vi "Telemetry_data_array_setup.vi"(8 "error in":errorcluster, 10 "Subsystem data":T1={"Subsystem name"="Drive", "Double data points"=[], "Boolean data points"=[], "Boolean channel names"=[], "Double channel names"=[]}, 11 "Channel & data arrays in":T2) -> (0 "error out":errorcluster, 3 "Channel & data arrays out":T2)   [LabVIEW 2017, in "labview-standard-library.lvlib" / "data-logging.lvlib"]
uses:
  data-logging.lvlib
  Channel&data_arrays.ctl
  Subsystem_data.ctl
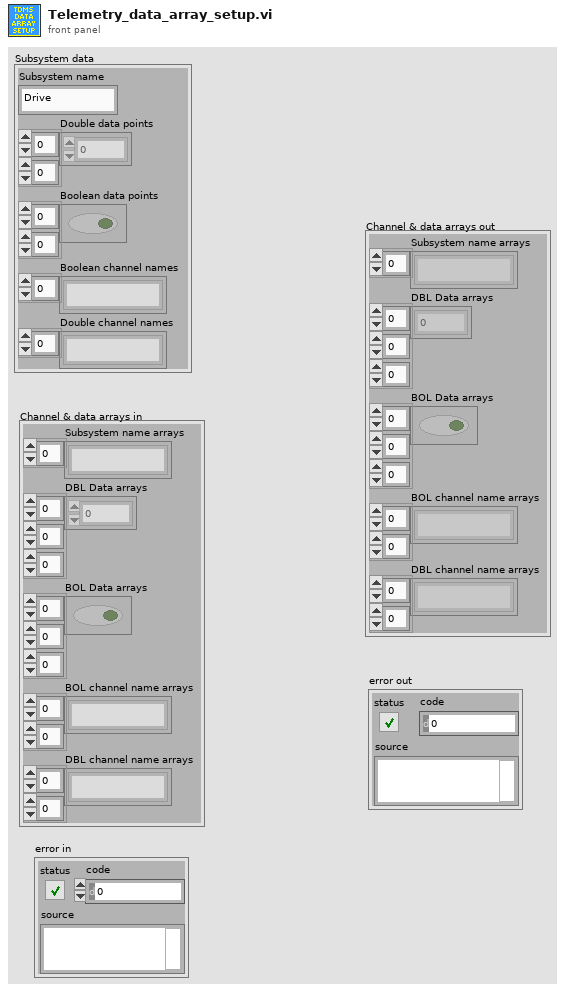
[diagram p1: front panel]
types:
  T1 = typedef "labview-standard-library.lvlib/data-logging.lvlib/Subsystem_data.ctl" = cluster{"Subsystem name":string, "Double data points":dbl[][], "Boolean data points":bool[][], "Boolean channel names":string[], "Double channel names":string[]}
  T2 = typedef "labview-standard-library.lvlib/data-logging.lvlib/Channel&data_arrays.ctl" = cluster{"Subsystem name arrays":string[], "DBL Data arrays":dbl[][][], "BOL Data arrays":bool[][][], "BOL channel name arrays":string[][], "DBL channel name arrays":string[][]}
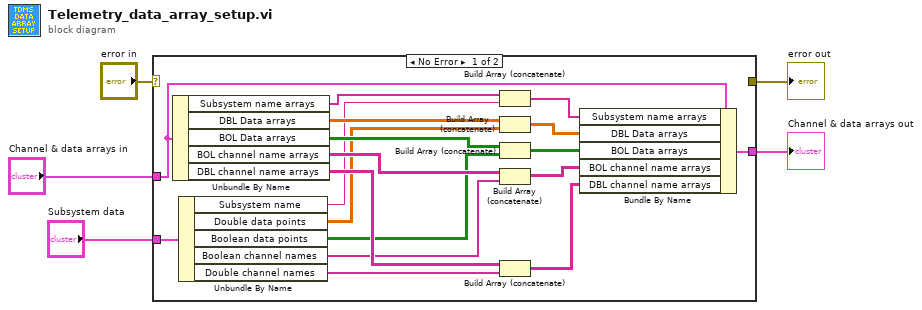
[diagram p0: block diagram]
diagram:
  n1 = case shown="No Error" "error in" {
    selector: "error in" -> [_ w24]
    tunnel: "Channel & data arrays in" -> [w12 w25]
    tunnel: [w13 w25] -> w4
    tunnel: [_ w24] -> w2
    tunnel: "Subsystem data" -> [w11 _]
    frame No Error {
      n2 = Unbundle By Name(w12) -> ("Subsystem name arrays"=w23:string[], "DBL Data arrays"=w22:dbl[][][], "BOL Data arrays"=w21:bool[][][], "BOL channel name arrays"=w20:string[][], "DBL channel name arrays"=w19:string[][])
      n3 = Unbundle By Name(w11) -> ("Subsystem name"=w10:string, "Double data points"=w9:dbl[][], "Boolean data points"=w8:bool[][], "Boolean channel names"=w7:string[], "Double channel names"=w6:string[])
      n4 = Build Array (concatenate)(w23, w10) -> (w18:string[])
      n5 = Build Array (concatenate)(w22, w9) -> (w17:dbl[][][])
      n6 = Build Array (concatenate)(w21, w8) -> (w16:bool[][][])
      n7 = Build Array (concatenate)(w20, w7) -> (w15:string[][])
      n8 = Build Array (concatenate)(w19, w6) -> (w14:string[][])
      n9 = Bundle By Name(cluster=w12, "Subsystem name arrays"=w18, "DBL Data arrays"=w17, "BOL Data arrays"=w16, "BOL channel name arrays"=w15, "DBL channel name arrays"=w14) -> (w13:T2)
    }
    frame Error {
    }
  }
  "Channel & data arrays out" <- w4
  "error out" <- w2
